vi "Ascii Symbol.vi"(11 "Character":u8) -> (3 "Symbol":T1, 5 "Open":bool)   [LabVIEW 2020]
uses:
  Open Symbol.ctl
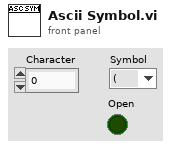
[diagram p1: front panel]
types:
  T1 = typedef "Open Symbol.ctl" = enum16{"(", "[", "{", "<"}
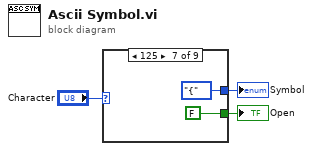
[diagram p0: block diagram]
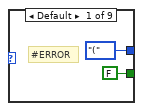
[diagram p2: hidden frame]
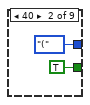
[diagram p3: hidden frame]
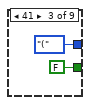
[diagram p4: hidden frame]
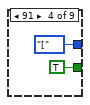
[diagram p5: hidden frame]
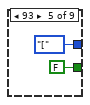
[diagram p6: hidden frame]
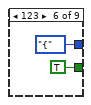
[diagram p7: hidden frame]
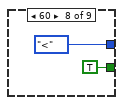
[diagram p8: hidden frame]
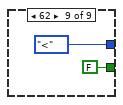
[diagram p9: hidden frame]
diagram:
  n1 = case shown="125" "Character" {
    tunnel: [Open_Symbol."(" ("Open Symbol") Open_Symbol."(" ("Open Symbol") Open_Symbol."(" ("Open Symbol") Open_Symbol."[" ("Open Symbol") Open_Symbol."[" ("Open Symbol") Open_Symbol."{" ("Open Symbol") Open_Symbol."{" ("Open Symbol") Open_Symbol."<" ("Open Symbol") Open_Symbol."<" ("Open Symbol")] -> w2
    tunnel: [FALSE TRUE FALSE TRUE FALSE TRUE FALSE TRUE FALSE] -> w1
    frame Default {
      # "#ERROR"
    }
    frame 40 {
    }
    frame 41 {
    }
    frame 91 {
    }
    frame 93 {
    }
    frame 123 {
    }
    frame 125 {
    }
    frame 60 {
    }
    frame 62 {
    }
  }
  "Symbol" <- w2
  "Open" <- w1
